vi "Delta_t.vi"() -> ()   [LabVIEW 2009]
panel:
  in  "dt":dbl
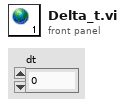
[diagram p1: front panel]
diagram:
